vi "Set Allow Debugging for VIs in Folder.vi"(8 "error in (no error)":errorcluster, 10 "Allow Debugging?":bool, 11 "VI Folder":path) -> (0 "error out":errorcluster, 3 "VI List":path[](array[path]))   [LabVIEW 2016, in "SLL Scripting.lvlib"]
doc: "This is used to set/unset the \"Allow Debugging\" option for all VIs in the specified folder."
uses:
  SLL Scripting.lvlib
panel:
  out "Progress":i32
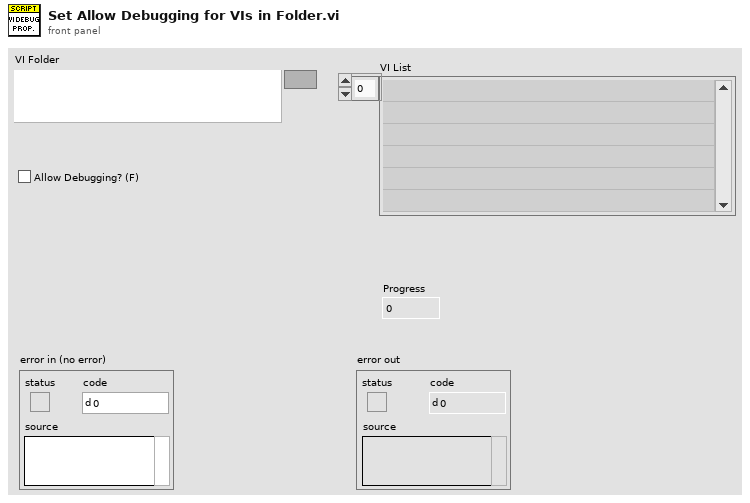
[diagram p1: front panel]
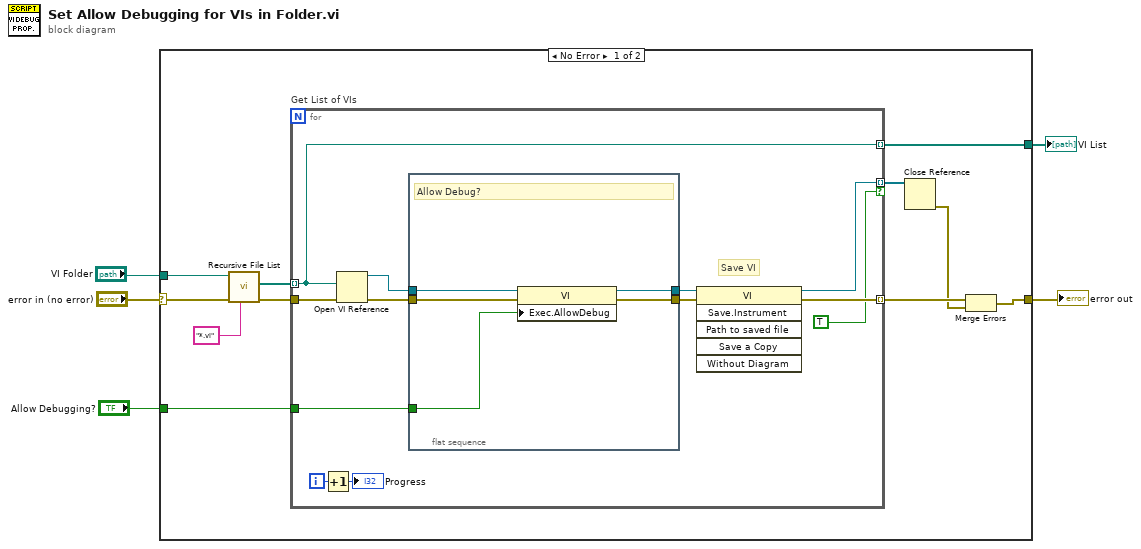
[diagram p0: block diagram]
diagram:
  n1 = case shown="No Error" "error in (no error)" {
    selector: "error in (no error)" -> [w11 w34]
    tunnel: "VI Folder" -> [w15 _]
    tunnel: [w12 _] -> w4
    tunnel: [w7 w34] -> w2
    tunnel: "Allow Debugging?" -> [w6 _]
    frame No Error {
      n2 = call <vilib>:"Recursive File List.vi"("pattern"="*.vi", "error in (no error)"=w11, "Folder Path"=w15) -> ("error out"=w10:errorcluster, "All Files in Dir"=w13:path[])  [unwired: 4 in, 3 out]
      n3 = for "Get List of VIs" {
        tunnel: [w26] -> w16 mode=indexing if=TRUE
        tunnel: w13 -> [w23] mode=indexing
        tunnel: [w23] -> w12 mode=indexing
        tunnel: w10 -> [w25]
        tunnel: [w27] -> w9 mode=indexing
        tunnel: w6 -> [w22]
        i -> [w28]
        # "Save VI"
        n4 = Increment(x=w28) -> (x+1=→"Progress":i32)
        n5 = Open VI Reference(vi path=w23, error in (no error)=w25) -> (vi reference=w21:refnum<vi>, error out=w20:errorcluster)  [unwired: 4 in]
        n6 = flat-sequence {
          tunnel: w21 -> [w31]
          tunnel: w20 -> [w33]
          tunnel: [w32] -> w19
          tunnel: [w30] -> w18
          tunnel: w22 -> [w29]
          frame #0 {
            # "Allow Debug?"
            n7 = property class="VI"(reference=w31, error in=w33, "Exec.AllowDebug"=w29) -> (reference out=w30:refnum<vi>, error out=w32:errorcluster)
          }
        }
        n8 = invoke class="VI" method="Save.Instrument"(reference=w18, error in=w19) -> (reference out=w26:refnum<vi>, error out=w27:errorcluster)  [unwired: 4 in, 4 out]
      }
      n9 = Close Reference(reference=w16) -> (error out=w8:errorcluster)  [unwired: 1 in]
      n10 = Merge Errors(w9, w8) -> (w7:errorcluster)
    }
    frame Error {
    }
  }
  "error out" <- w2
  "VI List" <- w4
